vi "Cam0 AprilTag Target Package.vi"(0 "Camera Name":string="cam0") -> ()   [LabVIEW 2023]
uses:
  <vilib>/vision/Shape Detection.llb/ShapeDetectionMatchOptions.ctl
  <vilib>/vision/Pattern Matching.llb/IMAQ Match Range Setting.ctl
  <vilib>/vision/Image Controls.llb/IMAQ Image.ctl
  Camera Set Up/Event Setup Types.ctl
  <vilib>/Rock Robotics/Network Tables/NT Write Numeric Array.vi
  <vilib>/Utility/config.llb/Write Key (String).vi
  <vilib>/Utility/config.llb/Read Key (String).vi
  <vilib>/Utility/config.llb/NI_LVConfig.lvlib
  <vilib>/vision/NI_Vision_Development_Module.lvlib
panel:
  in  "Main":enum32{"Page 1", "Page 2"}(tab)
  out "Image":T1(plugin-control)
  in  "Settings":bool
  in  "Save":bool
  in  "Tools":bool
  out "Fps":dbl format="%#.0f"
  in  "Target Size":dbl=6.5
  out "Distance":dbl[](array[numeric]) format="%.1f"
  out "Angle":dbl[](array[numeric]) format="%.1f"
  in  "Min Rect Size (pix)":dbl
  in  "Max Rect Size (pix)":dbl
  in  "Home":bool
  in  "Match Options":T2={"Rotation"=TRUE, "Scale"=TRUE, "Occlusion"=FALSE, "Range Settings"=[]} {"Range Settings"."Match Constraints" items=["Rotation Angle (degrees)", "Scale Factor (%)", "Occlusion (%)"]}
  in  "upper limit":sgl=1.2
  in  "lower limit":sgl=0.8
  # "Aspect Ratio"
  # "Range"
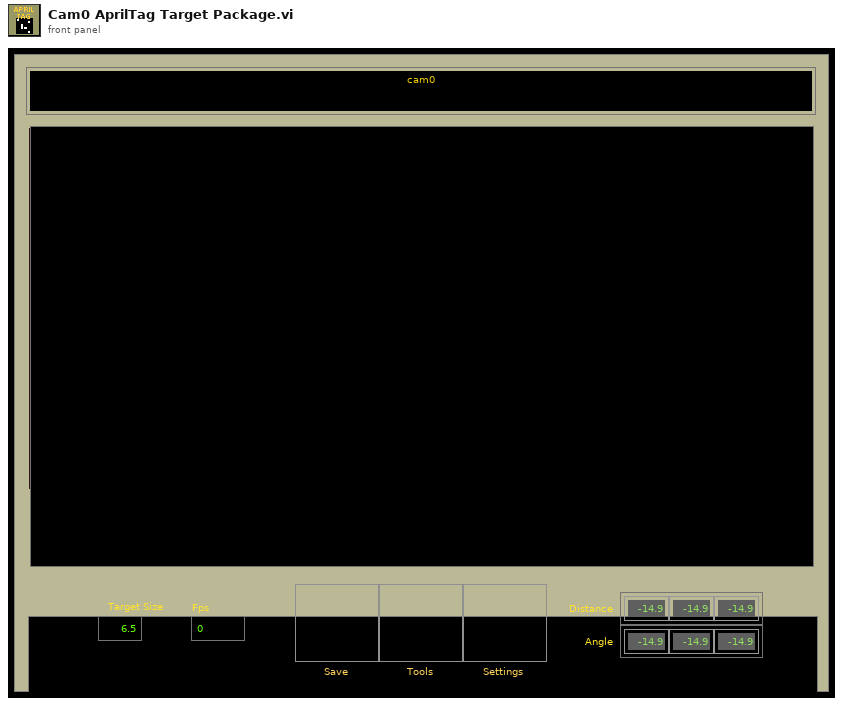
[diagram p1: front panel]
types:
  T1 = typedef "IMAQ Image.ctl" = refnum<image>
  T2 = typedef "ShapeDetectionMatchOptions.ctl" = cluster{"Rotation":bool, "Scale":bool, "Occlusion":bool, "Range Settings":T3[]}
  T3 = typedef "IMAQ Match Range Setting.ctl" = cluster{"Match Constraints":u32, "Min":dbl, "Max":dbl}
  T4 = typedef "Image Type" = u32
  T5 = cluster{"Min Width":dbl, "Max Width":dbl, "Min Height":dbl, "Max Height":dbl}
  T6 = typedef "Event Setup Types.ctl" = enum16{"Default", "Camera Loop Started", "Save Data", "Open Front Panel", "Exit"}
  T7 = cluster{"Corners":cluster{"X":sgl, "Y":sgl}[], "Angle":dbl, "Width":dbl, "Height":dbl, "Score":dbl}[]
  T8 = typedef "Target Fields.ctl" = cluster{"diameter points":cluster{"first point":cluster{"x":dbl, "y":dbl}, "projected point":cluster{"x":dbl, "y":dbl}}, "normalized center":cluster{"x":dbl, "y":dbl}, "Overall Score":dbl, "Area Score":dbl, "Moment Score":dbl, "Aspect Score":dbl, "Distance (ft)":dbl, "Upper Goal":bool}
  T9 = typedef "NI_LVConfig.lvlib/Config Data RefNum.ctl" = refnum<k1>
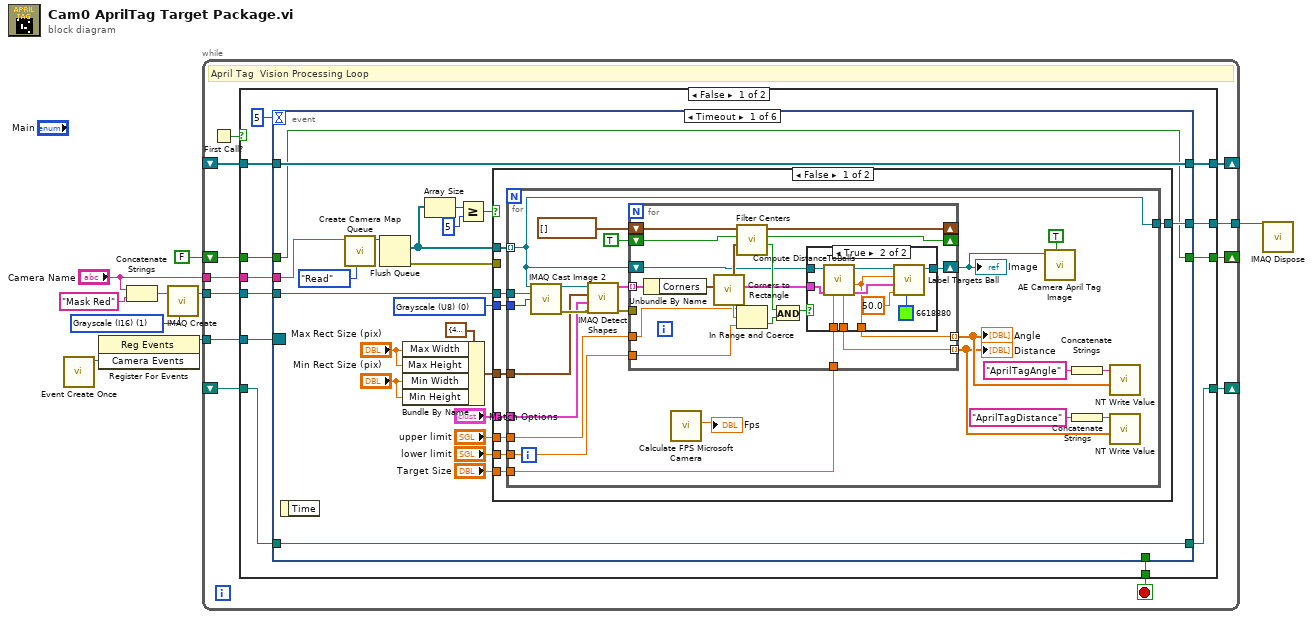
[diagram p0: block diagram]
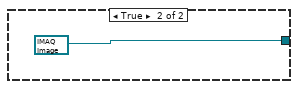
[diagram p3: hidden frame]
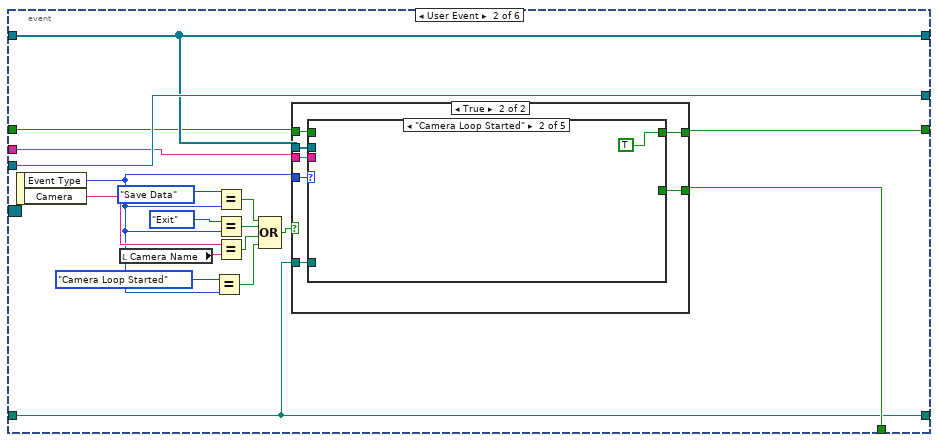
[diagram p4: hidden frame]
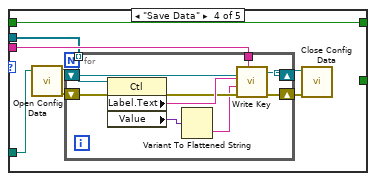
[diagram p8: hidden frame]
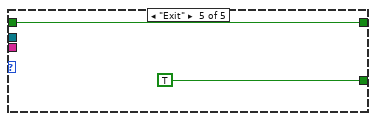
[diagram p9: hidden frame]
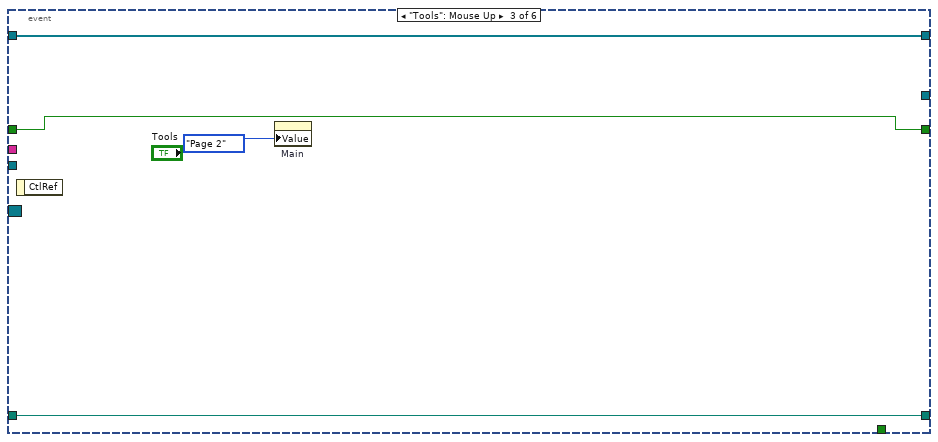
[diagram p10: hidden frame]
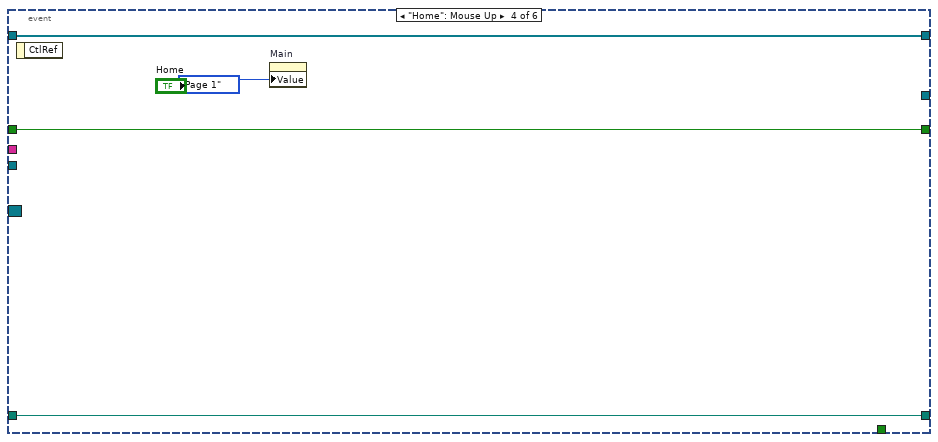
[diagram p11: hidden frame]
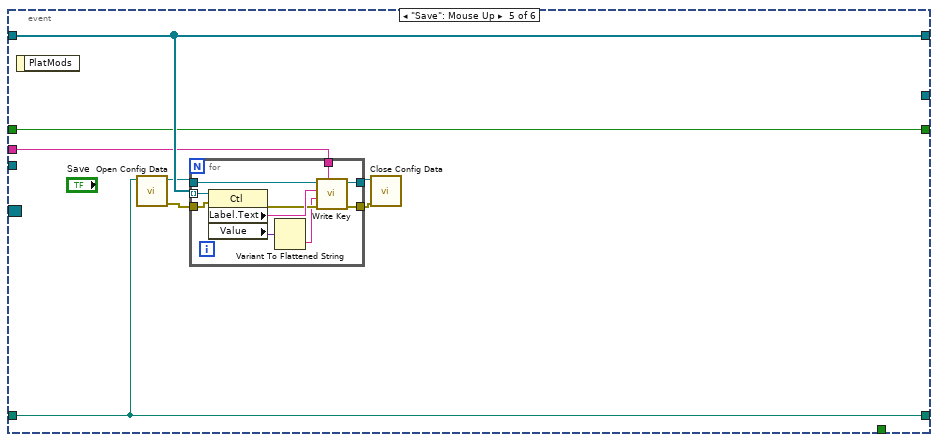
[diagram p12: hidden frame]
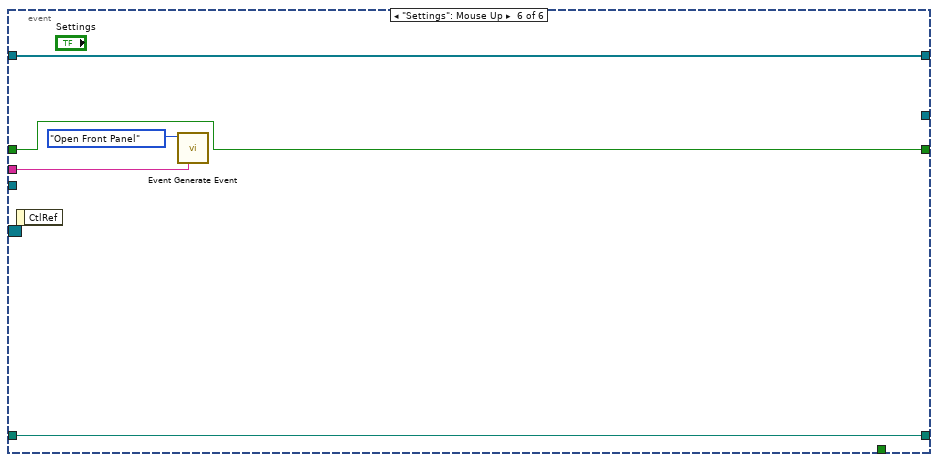
[diagram p13: hidden frame]
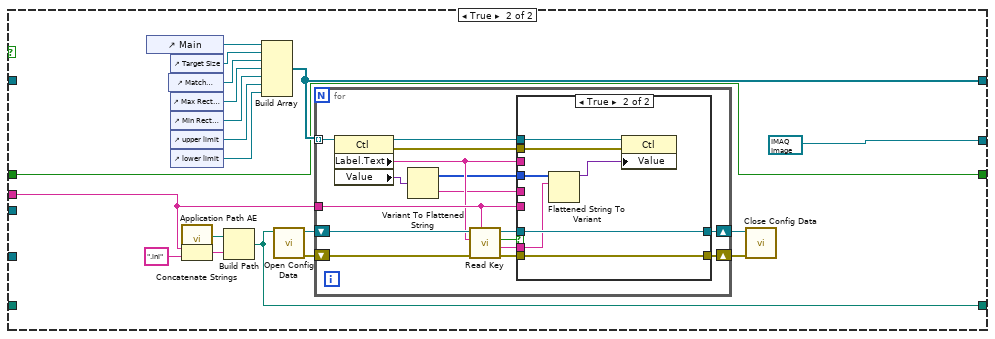
[diagram p14: hidden frame]
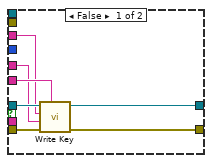
[diagram p15: hidden frame]
diagram:
  w6 = T4 1 items=["Grayscale (U8)", "Grayscale (I16)", "Grayscale (SGL)", "Complex (CSG)", "RGB (U32)", "HSL (U32)", "RGB (U64)", "Grayscale (U16)"] ("Image Type")
  n1 = call "Event Create Once.vi"() -> ("Camera Events"=w8:refnum<user-event>)  [unwired: 10 in, 1 out]
  n2 = register-events(w8) -> (reference out=w7:refnum<event-registration>)  [unwired: 2 in, 1 out]
  n3 = Concatenate Strings("Camera Name", "Mask Red" ("string")) -> (w5:string)
  n4 = call "IMAQ Create"("Image Name"=w5, "Image Type"=w6) -> ("New Image"=w9:T1)  [unwired: 2 in, 2 out]
  n5 = while {
    tunnel: w9 -> [w21]
    tunnel: [w20] -> w1
    tunnel: w7 -> [w19]
    tunnel: "Camera Name" -> [w17]
    shift-right: [w15] -> _
    shift-left: _ -> [w14]
    shift-right: [w13] -> _
    shift-left: _ -> [w12]
    shift-right: [w10] -> _
    shift-left: FALSE -> [w11]
    stop <- w18 stop-if-true
    # "April Tag  Vision Processing Loop"
    n6 = First Call?() -> (First Call?: T/F=w16:bool)
    n7 = case shown="False" w16 {
      tunnel: w21 -> [w33 _]
      tunnel: [w32 T1 refnum ("New Image")] -> w20
      tunnel: w19 -> [w31 _]
      tunnel: [w30 _] -> w18
      tunnel: w17 -> [w29 w211]
      tunnel: [w27 w207] -> w15
      tunnel: w14 -> [w28 _]
      tunnel: [w26 w210] -> w13
      tunnel: w12 -> [w24 _]
      tunnel: w11 -> [w23 w204]
      tunnel: [w22 w204] -> w10
      frame False {
        n8 = event shown="[0] Timeout" {
          selector: w31 -> [_ _ _ _ _ _]
          dyn-events: _ -> [_ _ _ _ _ _]
          timeout: 5 -> [_ _ _ _ _ _]
          tunnel: w33 -> [w54 w136 _ _ _ _]
          tunnel: [w55 w136 _ _ _ _] -> w32
          tunnel: [_ w135 _ _ _ _] -> w30
          tunnel: w29 -> [w51 w134 _ _ w179 w195]
          tunnel: w28 -> [w53 w132 w171 w175 w182 w198]
          tunnel: [w53 w132 w171 w175 w182 w198] -> w27
          tunnel: w24 -> [w52 w133 w170 w174 w183 w197]
          tunnel: [w52 w133 w170 w174 w183 w197] -> w26
          tunnel: w23 -> [w50 w123 w168 w172 w176 w194]
          tunnel: [w50 w122 w168 w172 w176 w194] -> w22
          event Timeout {
            w45 = T4 0 items=["Grayscale (U8)", "Grayscale (I16)", "Grayscale (SGL)", "Complex (CSG)", "RGB (U32)", "HSL (U32)", "RGB (U64)", "Grayscale (U16)"] ("Image Type")
            n9 = event-data() -> ()  [unwired: 1 in, 1 out]
            n10 = call "Create Camera Map Queue.vi"("Action"=enum16{"Read", "Write"}."Read", "Camera"=w51) -> ("value"=w47:refnum<queue>)  [unwired: 8 in, 1 out]
            n11 = Flush Queue(queue=w47) -> (remaining elements=w44:T1[], error out=w46:errorcluster)  [unwired: 1 in, 1 out]
            n12 = Bundle By Name(cluster=T5 {"Min Width"=40.0, "Max Width"=100.0, "Min Height"=40.0, "Max Height"=200.0} ("Rectangle Descriptor"), "Max Width"="Max Rect Size (pix)", "Max Height"="Max Rect Size (pix)", "Min Width"="Min Rect Size (pix)", "Min Height"="Min Rect Size (pix)") -> (w38:T5)
            n13 = Array Size(array=w44) -> (size(s)=w43:i32)
            n14 = Greater Or Equal?(x=w43, y=5) -> (x >= y?=w41:bool)
            n15 = case shown="False" w41 {
              tunnel: [w58 T1 refnum ("Image")] -> w55
              tunnel: w54 -> [w64 _]
              tunnel: "Target Size" -> [w63 _]
              tunnel: w44 -> [w62 _]
              tunnel: w46 -> [_ _]
              tunnel: w45 -> [w61 _]
              tunnel: w38 -> [w60 _]
              tunnel: "Match Options" -> [w59 _]
              tunnel: "lower limit" -> [w57 _]
              tunnel: "upper limit" -> [w56 _]
              frame False {
                n16 = for {
                  tunnel: w64 -> [w87]
                  tunnel: w62 -> [w77] mode=indexing
                  tunnel: w63 -> [w76]
                  tunnel: w61 -> [w86]
                  tunnel: w60 -> [w82]
                  tunnel: w59 -> [w81]
                  tunnel: [w77] -> w58
                  tunnel: w57 -> [w74]
                  tunnel: w56 -> [w73]
                  n17 = call "IMAQ Cast Image 2"("Image Src"=w77, "Image Dst"=w87, "Image Type"=w86) -> ("Image Dst Out"=w84:T1, "error out"=w83:errorcluster)  [unwired: 11 in]
                  n18 = call-poly "IMAQ Detect Shapes"("error in (no error)"=w83, "Match Options"=w81, "Rectangle Descriptor"=w82, "Image"=w84) -> ("error out"=w75:errorcluster, "Rectangles"=w78:T7)  [unwired: 5 in, 1 out]
                  n19 = for {
                    shift-right: [w88] -> w66
                    shift-left: w77 -> [w89]
                    shift-right: [w103] -> _
                    shift-left: cluster{"X":dbl, "Y":dbl}[] [] ("Centers 2") -> [w105]
                    shift-right: [w101] -> _
                    shift-left: TRUE -> [w102]
                    tunnel: w78 -> [w97] mode=indexing
                    tunnel: w76 -> [w94]
                    tunnel: [w93] -> w67 mode=indexing
                    tunnel: [w92] -> w69 mode=indexing
                    tunnel: w75 -> [_]
                    tunnel: w74 -> [w91]
                    tunnel: w73 -> [w90]
                    n20 = Unbundle By Name(w97) -> ("Corners"=w96:cluster{"X":sgl, "Y":sgl}[])
                    n21 = call "Corners to Rectangle.vi"("Corners 2"=w96) -> ("output cluster"=w95:T8, "Aspect Ratio"=w106:sgl, "Center"=w104:cluster{"X":dbl, "Y":dbl})  [unwired: 8 in]
                    n22 = call "Filter Centers.vi"("Center"=w104, "First time"=w102, "Centers"=w105) -> ("Added"=w100:bool, "First time Out"=w101:bool, "Centers 2"=w103:cluster{"X":dbl, "Y":dbl}[])  [unwired: 6 in]
                    n23 = In Range and Coerce(upper limit=w90, x=w106, lower limit=w91) -> (In Range?=w99:bool)  [unwired: 1 out]
                    n24 = And(x=w100, y=w99) -> (x .and. y?=w98:bool)
                    n25 = case shown="True" w98 {
                      tunnel: w89 -> [w107 w116]
                      tunnel: [w107 w117] -> w88
                      tunnel: w95 -> [_ w111]
                      tunnel: w94 -> [_ w110]
                      tunnel: [_ w109] -> w93
                      tunnel: [_ w108] -> w92
                      frame False {
                      }
                      frame True {
                        n26 = call "Compute DistanceToBalls.vi"("Target Width (in)"=w110, "results"=w111, "Image Src"=w116) -> ("results out"=w112:T8, "Off Angle"=w108:dbl, "Image Dst Out"=w114:T1, "Distance"=w109:dbl)  [unwired: 4 in, 1 out]
                        n27 = call "Label Targets Ball.vi"("Color"=u32 6618880, "Score Threshold"=50.0, "results"=w112, "Angle"=w108, "Image in"=w114) -> ("Image out"=w117:T1)  [unwired: 6 in]
                      }
                    }
                  }
                  "Image" <- w66
                  "Angle" <- w69
                  "Distance" <- w67
                  n28 = call "Calculate FPS Microsoft Camera.vi"() -> ("Fps"=→"Fps":dbl)  [unwired: 11 in]
                  n29 = call "AE Camera April Tag Image.vi"("Update"=TRUE, "Ball Image in"=w66) -> ()  [unwired: 9 in, 1 out]
                  n30 = Concatenate Strings("AprilTagAngle" ("Name")) -> (w68:string)
                  n31 = Concatenate Strings("AprilTagDistance" ("Name")) -> (w72:string)
                  n32 = call-poly <vilib>:"NT Write Value.vi"("value"=w69, "name"=w68) -> ()  [unwired: 9 in, 1 out]
                  n33 = call-poly <vilib>:"NT Write Value.vi"("value"=w67, "name"=w72) -> ()  [unwired: 9 in, 1 out]
                }
              }
              frame True {
              }
            }
          }
          event User Event {
            n34 = event-data() -> ("Event Type"=w121:T6, "Camera"=w126:string)  [unwired: 1 in]
            n35 = local read "Camera Name"() -> (w127:string)
            n36 = Equal?(x=Event_Setup_Types."Camera Loop Started", y=w121) -> (x = y?=w119:bool)
            n37 = Equal?(x=Event_Setup_Types."Save Data", y=w121) -> (x = y?=w128:bool)
            n38 = Equal?(x=Event_Setup_Types."Exit", y=w121) -> (x = y?=w130:bool)
            n39 = Equal?(x=w126, y=w127) -> (x = y?=w125:bool)
            n40 = Compound Arithmetic op=OR(w128, w130, w125, w119) -> (w124:bool)
            n41 = case shown="True" w124 {
              tunnel: w121 -> [_ w144]
              tunnel: [_ w143] -> w135
              tunnel: w134 -> [_ w142]
              tunnel: w133 -> [_ w141]
              tunnel: w132 -> [_ w140]
              tunnel: w123 -> [w137 w139]
              tunnel: [w137 w138] -> w122
              frame False {
              }
              frame True {
                n42 = case shown="\"Camera Loop Started\"" w144 {
                  tunnel: [_ _ _ _ TRUE] -> w143
                  tunnel: w142 -> [_ _ _ w151 _]
                  tunnel: w141 -> [_ _ _ w150 _]
                  tunnel: w140 -> [_ _ _ w149 _]
                  tunnel: w139 -> [w145 _ w147 w148 w166]
                  tunnel: [w145 TRUE w147 w148 w166] -> w138
                  frame "Default" {
                  }
                  frame "Camera Loop Started" {
                  }
                  frame "Open Front Panel" {
                  }
                  frame "Save Data" {
                    n43 = call <vilib>:"Open Config Data.vi"("configuration file path"=w150) -> ("error out"=w152:errorcluster, "refnum"=w155:T9)  [unwired: 8 in, 1 out]
                    n44 = for {
                      tunnel: w151 -> [w161]
                      tunnel: w149 -> [w160] mode=indexing
                      shift-right: [w164] -> w154
                      shift-left: w155 -> [w165]
                      shift-right: [w163] -> w153
                      shift-left: w152 -> [w162]
                      n45 = property class="Ctl"(reference=w160, error in=w162) -> (error out=w157:errorcluster, "Label.Text"=w159:string, "Value"=w158:variant)  [unwired: 1 out]
                      n46 = Variant To Flattened String(Variant=w158) -> (data string=w156:string)  [unwired: 1 out]
                      n47 = call-poly <vilib>:"Write Key.vi"("section"=w161, "error in (no error)"=w157, "value"=w156, "key"=w159, "refnum"=w165) -> ("error out"=w163:errorcluster, "refnum out"=w164:T9)  [unwired: 4 in, 1 out]
                    }
                    n48 = call <vilib>:"Close Config Data.vi"("error in (no error)"=w153, "refnum"=w154) -> ()  [unwired: 8 in, 2 out]
                  }
                  frame "Exit" {
                  }
                }
              }
            }
          }
          event "Tools": Mouse Up {
            n49 = event-data() -> ()  [unwired: 1 in, 1 out]
            n50 = property on="Main" class="TabCtl (strict)"("Value"=enum32{"Page 1", "Page 2"}."Page 2" ("Main")) -> ()  [unwired: 2 in, 2 out]
          }
          event "Home": Mouse Up {
            n51 = event-data() -> ()  [unwired: 1 in, 1 out]
            n52 = property on="Main" class="TabCtl (strict)"("Value"=enum32{"Page 1", "Page 2"}."Page 1" ("Main")) -> ()  [unwired: 2 in, 2 out]
          }
          event "Save": Mouse Up {
            n53 = event-data() -> ()  [unwired: 1 in, 1 out]
            n54 = call <vilib>:"Open Config Data.vi"("configuration file path"=w183) -> ("error out"=w180:errorcluster, "refnum"=w181:T9)  [unwired: 8 in, 1 out]
            n55 = for {
              tunnel: w182 -> [w193] mode=indexing
              tunnel: w181 -> [w192]
              tunnel: w180 -> [w191]
              tunnel: w179 -> [w187]
              tunnel: [w185] -> w178
              tunnel: [w184] -> w177
              n56 = property class="Ctl"(reference=w193, error in=w191) -> (error out=w188:errorcluster, "Label.Text"=w190:string, "Value"=w189:variant)  [unwired: 1 out]
              n57 = Variant To Flattened String(Variant=w189) -> (data string=w186:string)  [unwired: 1 out]
              n58 = call-poly <vilib>:"Write Key.vi"("section"=w187, "error in (no error)"=w188, "value"=w186, "key"=w190, "refnum"=w192) -> ("error out"=w185:errorcluster, "refnum out"=w184:T9)  [unwired: 4 in, 1 out]
            }
            n59 = call <vilib>:"Close Config Data.vi"("error in (no error)"=w178, "refnum"=w177) -> ()  [unwired: 8 in, 2 out]
          }
          event "Settings": Mouse Up {
            n60 = event-data() -> ()  [unwired: 1 in, 1 out]
            n61 = call "Event Generate Event.vi"("Camera Name"=w195, "Event Type"=Event_Setup_Types."Open Front Panel") -> ()  [unwired: 10 in]
          }
        }
      }
      frame True {
        n62 = control-ref of="Main"() -> (w206:refnum<vi>)
        n63 = control-ref of="Match Options"() -> (w203:refnum<vi>)
        n64 = control-ref of="Target Size"() -> (w205:refnum<vi>)
        n65 = control-ref of="Max Rect Size (pix)"() -> (w202:refnum<vi>)
        n66 = control-ref of="Min Rect Size (pix)"() -> (w201:refnum<vi>)
        n67 = control-ref of="upper limit"() -> (w200:refnum<vi>)
        n68 = control-ref of="lower limit"() -> (w199:refnum<vi>)
        n69 = call "Application Path AE.vi"() -> ("Application Path out"=w208:path)  [unwired: 11 in]
        n70 = Concatenate Strings(w211, ".ini" ("name or relative path")) -> (w216:string)
        n71 = Build Path(base path=w208, name or relative path=w216) -> (appended path=w210:path)
        n72 = Build Array(w206, w205, w203, w202, w201, w200, w199) -> (w207:refnum<vi>[])
        n73 = call <vilib>:"Open Config Data.vi"("configuration file path"=w210) -> ("error out"=w209:errorcluster, "refnum"=w215:T9)  [unwired: 8 in, 1 out]
        n74 = for {
          tunnel: w211 -> [w230]
          tunnel: w207 -> [w220] mode=indexing
          shift-right: [w232] -> w214
          shift-left: w215 -> [w233]
          shift-right: [w231] -> w213
          shift-left: w209 -> [w229]
          n75 = property class="Ctl"(reference=w220) -> (reference out=w226:refnum<vi>, error out=w225:errorcluster, "Label.Text"=w223:string, "Value"=w219:variant)  [unwired: 1 in]
          n76 = Variant To Flattened String(Variant=w219) -> (data string=w221:string, 1:w218:i16[])
          n77 = call-poly <vilib>:"Read Key.vi"("section"=w230, "error in (no error)"=w229, "key"=w223, "refnum"=w233) -> ("error out"=w222:errorcluster, "value"=w227:string, "found?"=w228:bool, "refnum out"=w224:T9)  [unwired: 4 in]
          n78 = case shown="True" w228 {
            tunnel: w227 -> [_ w242]
            tunnel: w226 -> [_ w247]
            tunnel: w225 -> [_ w246]
            tunnel: w224 -> [w240 w245]
            tunnel: w230 -> [w239 _]
            tunnel: w223 -> [w238 _]
            tunnel: [w237 w245] -> w232
            tunnel: w222 -> [w236 w244]
            tunnel: [w235 w244] -> w231
            tunnel: w221 -> [w234 _]
            tunnel: w218 -> [_ w241]
            frame False {
              n79 = call-poly <vilib>:"Write Key.vi"("section"=w239, "error in (no error)"=w236, "value"=w234, "key"=w238, "refnum"=w240) -> ("error out"=w235:errorcluster, "refnum out"=w237:T9)  [unwired: 4 in, 1 out]
            }
            frame True {
              n80 = Flattened String To Variant(6:w242, 7:w241) -> (3:w243:variant)  [unwired: 1 in, 1 out]
              n81 = property class="Ctl"(reference=w247, error in=w246, "Value"=w243) -> ()  [unwired: 2 out]
            }
          }
        }
        n82 = call <vilib>:"Close Config Data.vi"("error in (no error)"=w213, "refnum"=w214) -> ()  [unwired: 8 in, 2 out]
      }
    }
  }
  n83 = call "IMAQ Dispose"("Image"=w1) -> ()  [unwired: 5 in, 1 out]
